vi "RPI2 Expand File System.vi"(8 "Error In":errorcluster, 11 "Install LV Data":T1={"SSH Session"=refnum, "Status Log"="", "Detailed Log"="", "Credentials"={"Hostname or IP"="192.168.7.2", "Username"="root", "Password"=""}, "Target Info"={"OS Version"="", "CPU"="", "Systemd Version"="", "Internet Access"=FALSE, "Device Type"="", "LV Installed Ver"="", "LV Available Ver"="", "LV Upgrade Available"=FALSE, "Hostname"="", "NIC Info"=[]}, "Reboot Required?"=FALSE}) -> (0 "Error Out":errorcluster, 2 "Fixed?":bool, 3 "Install LV Data":T1={"SSH Session"=refnum, "Status Log"="", "Detailed Log"="", "Credentials"={"Hostname or IP"="192.168.7.2", "Username"="root", "Password"=""}, "Target Info"={"OS Version"="", "CPU"="", "Systemd Version"="", "Internet Access"=FALSE, "Device Type"="", "LV Installed Ver"="", "LV Available Ver"="", "LV Upgrade Available"=FALSE, "Hostname"="", "NIC Info"=[]}, "Reboot Required?"=FALSE})   [LabVIEW 2020, in "LMH-LINX.lvlib"]
uses:
  LMH-LINX.lvlib
  Install LV Data.ctl
  Target Info.ctl
  NIC Info.ctl
  NIC Mode.ctl
  Status FGV States.ctl
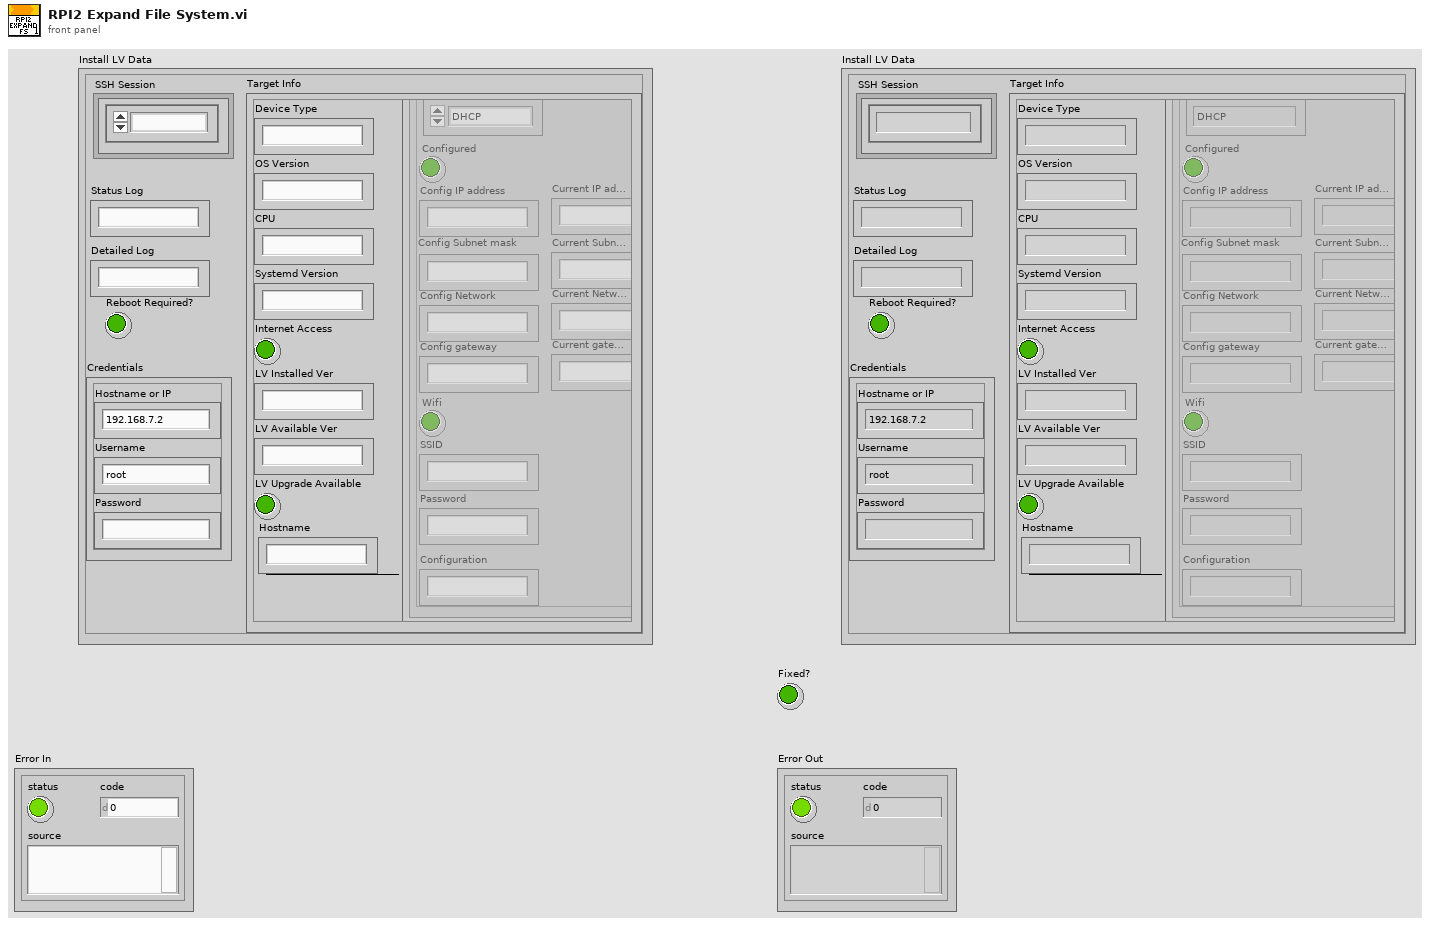
[diagram p1: front panel]
types:
  T1 = typedef "LMH-LINX.lvlib/Install LV Data.ctl" = cluster{"SSH Session":refnum<k1>, "Status Log":string, "Detailed Log":string, "Credentials":cluster{"Hostname or IP":string, "Username":string, "Password":string}, "Target Info":T2, "Reboot Required?":bool}
  T2 = typedef "LMH-LINX.lvlib/Target Info.ctl" = cluster{"OS Version":string, "CPU":string, "Systemd Version":string, "Internet Access":bool, "Device Type":string, "LV Installed Ver":string, "LV Available Ver":string, "LV Upgrade Available":bool, "Hostname":string, "NIC Info":T3[]}
  T3 = typedef "LMH-LINX.lvlib/NIC Info.ctl" = cluster{"Name":string, "NIC Mode":T4, "Configured":bool, "Config IP address":string, "Config Subnet mask":string, "Config Network":string, "Config gateway":string, "Wifi":bool, "SSID":string, "Password":string, "Configuration":string, "Current IP address":string, "Current Subnet mask":string, "Current gateway":string, "Current Network":string}
  T4 = typedef "LMH-LINX.lvlib/NIC Mode.ctl" = enum16{"DHCP", "Static", "Loopback"}
  T5 = typedef "LMH-LINX.lvlib/Status FGV States.ctl" = enum16{"Init", "Append", "Append History Only", "Set", "Get"}
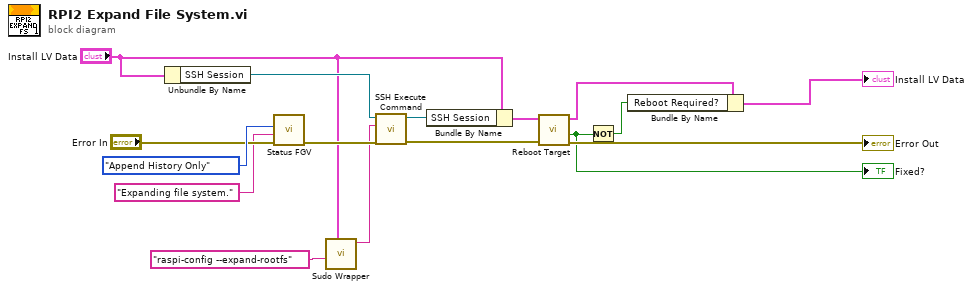
[diagram p0: block diagram]
diagram:
  n1 = Unbundle By Name("Install LV Data") -> ("SSH Session"=w7:refnum<k1>)
  n2 = call "Status FGV.vi"("Error In"="Error In", "Status"="Expanding file system.", "Status FGV State"=Status_FGV_States."Append History Only") -> ("Error Out"=w9:errorcluster)  [unwired: 6 in, 2 out]
  n3 = call "Sudo Wrapper.vi"("Install LV Data"="Install LV Data", "comand string"="raspi-config --expand-rootfs" ("Command")) -> ("combined command string"=w2:string)  [unwired: 9 in]
  n4 = call "SSH Execute Command.vi"("Error In"=w9, "Command"=w2, "SSH Session"=w7) -> ("Error Out"=w8:errorcluster, "SSH Session"=w6:refnum<k1>)  [unwired: 6 in, 1 out]
  n5 = Bundle By Name(cluster="Install LV Data", "SSH Session"=w6) -> (w5:T1)
  n6 = call "Reboot Target.vi"("Error In"=w8, "Install LV Data"=w5) -> ("Error Out"=→"Error Out":errorcluster, "Connected?"=w4:bool, "Install LV Data"=w13:T1)  [unwired: 7 in]
  "Fixed?" <- w4
  n7 = Not(x=w4) -> (.not. x?=w11:bool)
  n8 = Bundle By Name(cluster=w13, "Reboot Required?"=w11) -> (→"Install LV Data":T1)
